vi "DrawCursorLinesFromMem.vi"(7 "CursorMode":bool, 8 "RedPositionArray":dbl[][](array[numeric]), 9 "BluePositionArray":dbl[][](array[numeric]), 10 "Red":refnum<vi>, 11 "Blue":refnum<vi>) -> ()   [LabVIEW 2013, in "main.lvlib"]
uses:
  main.lvlib
  Controls/Enum Variables.ctl
panel:
  in  "empty picture":picture
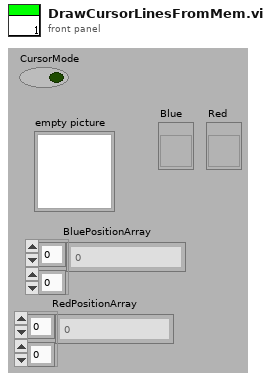
[diagram p1: front panel]
types:
  T1 = typedef "main.lvlib/Enum Variables.ctl" = enum16{"SetAcqFilter", "GetAcqFilter", "Set Filter", "Get Filter", "Set Height", "Get Height", "Set Recorded Height", "Get Recorded Height", "Set Blue Pressure", "Get Blue Pressure", "Set Red Pressure", "Get Red Pressure", "Init", "Reset Pressure", "Set Red Cursors", "Get Red Cursors", "Set Blue Cursors", "Get Blue Cursors", "Set Language", "Get Language", "Set Active Graphs", "Get ActiveGraphs", "Set Method", "Get Method", "Set Encryption", "Get Encryption", "Set ExcelVersion", "Get ExcelVersion", "Set DICOM Avail", "Get DICOM Avail", "Set DICOM Encode", "Get DICOM Encode", "Set JournalExport", "Get JournalExport", "Set Sequence", "Get Sequence", "Set DAQ Connected", "Get DAQ Connected", "Set Current Graph", "Get Current Graph", "Set General Settings", "Get Hyphenation", "Set Arm Calc Method", "Get Arm Calc Method", "Set Dicom Tags", "Get Dicom Tags", "Set BT Serial", "Get BT Serial", "Set BT Accepted Serials", "Get BT Accepted Serials", "Get BT License", "Set BT License"}
  T2 = cluster{"Width":u16, "Style":enum32{"Solid", "Dash", "Dot", "DashDot", "DashDotDot"}}
  T3 = typedef "LVRectTypeDef.ctl" = cluster{"Left":i16, "Top":i16, "Right":i16, "Bottom":i16}
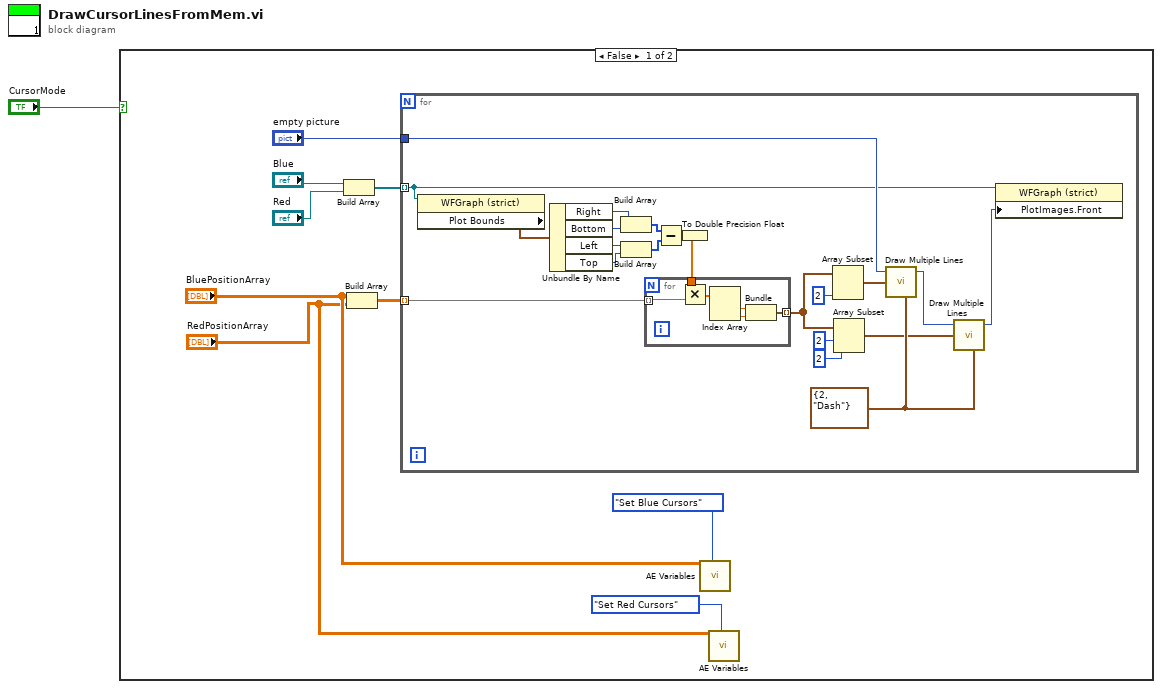
[diagram p0: block diagram]
diagram:
  n1 = case shown="False" "CursorMode" {
    frame False {
      n2 = Build Array("Blue", "Red") -> (w7:refnum<vi>[])
      n3 = Build Array("BluePositionArray", "RedPositionArray") -> (w6:dbl[][][])
      n4 = for {
        tunnel: "empty picture" -> [w24]
        tunnel: w6 -> [w22] mode=indexing
        tunnel: w7 -> [w20] mode=indexing
        w31 = T2 {"Width"=2, "Style"=enum."Dash"} ("pen")
        n5 = property class="WFGraph (strict)"(reference=w20) -> ("Plot Bounds"=w19:T3)  [unwired: 1 in, 2 out]
        n6 = Unbundle By Name(w19) -> ("Right"=w18:i16, "Bottom"=w17:i16, "Left"=w15:i16, "Top"=w14:i16)
        n7 = Build Array(w18, w17) -> (w13:i16[])
        n8 = Build Array(w15, w14) -> (w12:i16[])
        n9 = Subtract(x=w13, y=w12) -> (x-y=w11:i16[])
        n10 = To Double Precision Float(number=w11) -> (double precision float=w16:dbl[])
        n11 = for {
          tunnel: w22 -> [w33] mode=indexing
          tunnel: [w35] -> w21 mode=indexing
          tunnel: w16 -> [w32]
          n12 = Multiply(x=w32, y=w33) -> (x*y=w34:dbl[])
          n13 = Index Array(array=w34) -> (element #1=w37:dbl, element #2=w36:dbl)  [unwired: 2 in]
          n14 = Bundle(w37, w36) -> (w35:cluster{dbl, dbl})  [unwired: 1 in]
        }
        n15 = Array Subset(array=w21, length=2) -> (w26:cluster{dbl, dbl}[])  [unwired: 1 in]
        n16 = Array Subset(array=w21, index=2, length=2) -> (w29:cluster{dbl, dbl}[])
        n17 = call <vilib>:"Draw Multiple Lines.vi"("picture"=w24, "line endpoints"=w26, "pen"=w31) -> ("new picture"=w30:picture)  [unwired: 6 in]
        n18 = call <vilib>:"Draw Multiple Lines.vi"("picture"=w30, "line endpoints"=w29, "pen"=w31) -> ("new picture"=w23:picture)  [unwired: 6 in]
        n19 = property class="WFGraph (strict)"(reference=w20, "PlotImages.Front"=w23) -> ()  [unwired: 1 in, 2 out]
      }
      n20 = call "AE Variables.vi"("VariantIn"="BluePositionArray", "Action"=Enum_Variables."Set Blue Cursors") -> ()  [unwired: 10 in, 8 out]
      n21 = call "AE Variables.vi"("VariantIn"="RedPositionArray", "Action"=Enum_Variables."Set Red Cursors") -> ()  [unwired: 10 in, 8 out]
    }
    frame True {
    }
  }
